vi "cksum (SubVI).vi"(11 "Input String":string) -> (3 "Checksum":string)   [LabVIEW 2013]
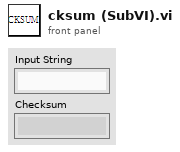
[diagram p1: front panel]
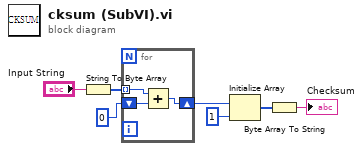
[diagram p0: block diagram]
diagram:
  n1 = String To Byte Array(string="Input String") -> (unsigned byte array=w6:u8[])
  n2 = for {
    tunnel: w6 -> [w10] mode=indexing
    shift-right: [w8] -> w3
    shift-left: u8 0 -> [w9]
    n3 = Add(x=w10, y=w9) -> (x+y=w8:u8)
  }
  n4 = Initialize Array(w3, 1 ("dimension size")) -> (w5:u8[])
  n5 = Byte Array To String(unsigned byte array=w5) -> (string=→"Checksum":string)
